vi "HAL process.vi"   [LabVIEW 2016]
uses:
  <vilib>/Plasmionique/MB Master/MB_Master/MB_Master.lvclass
  PLC/PLC.lvlib
types:
  T1 = cluster{"SYSTEM Interface":cluster{"运行模式":enum16{"维护模式", "常规模式", "应急模式", "质控模式"}, "站点类型":enum16{"一体站", "固定站"}, "CODMn类型":enum16{"PLC版", "单片机版"}, "总磷总氮类型":enum16{"单模块", "二合一模块"}}, "Pump Interface":cluster{"Pump MB session in":refnum<class "MB_Master.lvclass">}, "NH3N Interface":cluster{"NH3N session in":refnum<class "MB_Master.lvclass">, "氨氮自动测试量程配置":cluster{"水样测试量程模式":enum16{"H", "L", "AUTO"}, "空白核查量程模式":enum16{"H", "L", "AUTO"}, "跨度核查量程模式":enum16{"H", "L", "AUTO"}, "加标回收量程模式":enum16{"H", "L", "AUTO"}}}, "TP Interface":cluster{"TP MB session in":refnum<class "MB_Master.lvclass">, "总磷自动测试量程配置":cluster{"水样测试量程模式":enum16{"H", "L", "AUTO"}, "空白核查量程模式":enum16{"H", "L", "AUTO"}, "跨度核查量程模式":enum16{"H", "L", "AUTO"}, "加标回收量程模式":enum16{"H", "L", "AUTO"}}}, "TN Interface":cluster{"TN MB session in":refnum<class "MB_Master.lvclass">, "总氮自动测试量程配置":cluster{"水样测试量程模式":enum16{"H", "L", "AUTO"}, "空白核查量程模式":enum16{"H", "L", "AUTO"}, "跨度核查量程模式":enum16{"H", "L", "AUTO"}, "加标回收量程模式":enum16{"H", "L", "AUTO"}}}, "CODMn Interface":cluster{"CODMn MB session in":refnum<class "MB_Master.lvclass">, "CODMn自动测试量程配置":cluster{"水样测试量程模式":enum16{"H", "L", "AUTO"}, "空白核查量程模式":enum16{"H", "L", "AUTO"}, "跨度核查量程模式":enum16{"H", "L", "AUTO"}, "加标回收量程模式":enum16{"H", "L", "AUTO"}}}, "CODCr Interface":cluster{"CODCr MB session in":refnum<class "MB_Master.lvclass">, "CODCr自动测试量程配置":cluster{"水样测试量程模式":enum16{"H", "L", "AUTO"}, "空白核查量程模式":enum16{"H", "L", "AUTO"}, "跨度核查量程模式":enum16{"H", "L", "AUTO"}, "加标回收量程模式":enum16{"H", "L", "AUTO"}}}, "PLC_CODMn Interface":cluster{"PLC版_CODMn状态":u16, "PLC版_CODMn测量数据区":cluster{"因子编码":u32, "单位":u16, "标样参考值":sgl, "水样数据时间":timestamp, "水样实测值":sgl, "水样数据标识":string, "标样数据时间":timestamp, "标样实测值":sgl, "标样数据标识":string, "空白数据时间":timestamp, "空白实测值":sgl, "空白数据标识":string, "零点核查数据时间":timestamp, "零点核查实测值":sgl, "零点核查数据标识":string, "跨度核查数据时间":timestamp, "跨度核查实测值":sgl, "跨度核查数据标识":string, "加标回收数据时间":timestamp, "加标回收实测值":sgl, "加标回收数据标识":string, "平行样数据时间":timestamp, "平行样实测值":sgl, "平行样数据标识":string}}}
  T2 = cluster{"水样测试量程模式":enum16{"H", "L", "AUTO"}, "空白核查量程模式":enum16{"H", "L", "AUTO"}, "跨度核查量程模式":enum16{"H", "L", "AUTO"}, "加标回收量程模式":enum16{"H", "L", "AUTO"}}
  T3 = cluster{"水样测试量程模式":enum16{"H", "L", "AUTO"}, "空白核查量程模式":enum16{"H", "L", "AUTO"}, "跨度核查量程模式":enum16{"H", "L", "AUTO"}, "加标回收量程模式":enum16{"H", "L", "AUTO"}, "标样核查量程模式":enum16{"H", "L", "AUTO"}}
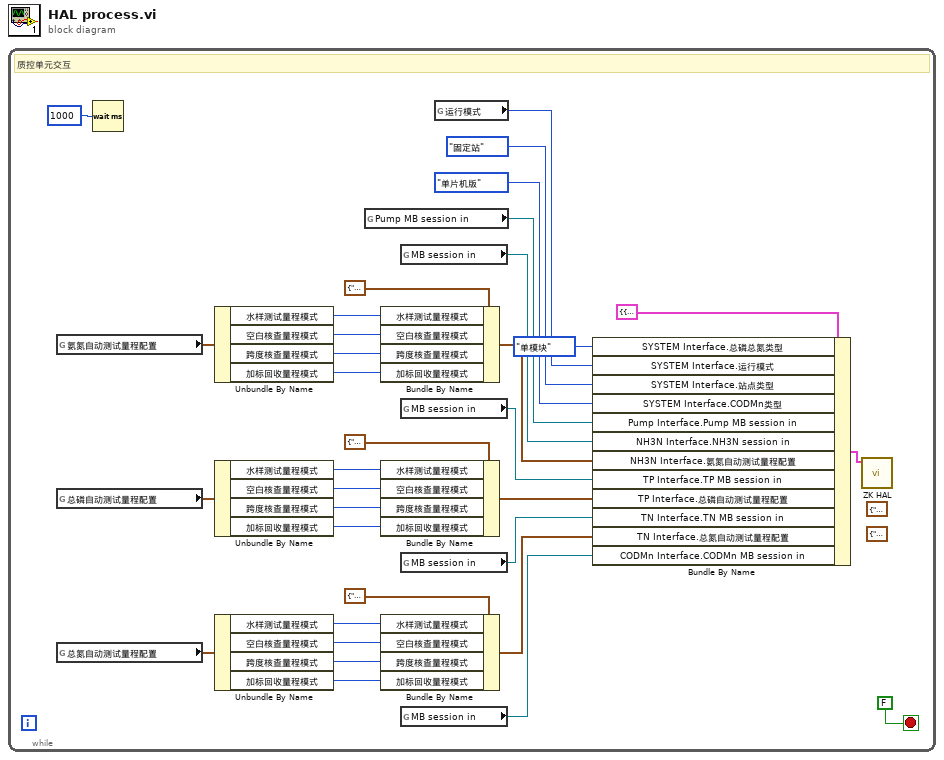
[diagram p0: block diagram]
diagram:
  n1 = while {
    stop <- FALSE stop-if-true
    (unwired) T2 {"水样测试量程模式"=enum."H", "空白核查量程模式"=enum."H", "跨度核查量程模式"=enum."H", "加标回收量程模式"=enum."H"} ("NH3N Interface.氨氮自动测试量程配置")
    (unwired) T2 {"水样测试量程模式"=enum."H", "空白核查量程模式"=enum."H", "跨度核查量程模式"=enum."H", "加标回收量程模式"=enum."H"} ("NH3N Interface.氨氮自动测试量程配置")
    # "质控单元交互"
    n2 = global read "总磷总氮断电保存全局变量.vi" "氨氮自动测试量程配置"() -> (w22:T3)
    n3 = global read "总磷总氮断电保存全局变量.vi" "总磷自动测试量程配置"() -> (w17:T3)
    n4 = global read "总磷总氮断电保存全局变量.vi" "总氮自动测试量程配置"() -> (w16:T3)
    n5 = Wait (ms)(milliseconds to wait=u32 1000 ("等待时间（毫秒）")) -> ()  [unwired: 1 out]
    n6 = Unbundle By Name(w22) -> ("水样测试量程模式"=w21:enum16{"H", "L", "AUTO"}, "空白核查量程模式"=w20:enum16{"H", "L", "AUTO"}, "跨度核查量程模式"=w19:enum16{"H", "L", "AUTO"}, "加标回收量程模式"=w18:enum16{"H", "L", "AUTO"})
    n7 = Unbundle By Name(w17) -> ("水样测试量程模式"=w13:enum16{"H", "L", "AUTO"}, "空白核查量程模式"=w12:enum16{"H", "L", "AUTO"}, "跨度核查量程模式"=w11:enum16{"H", "L", "AUTO"}, "加标回收量程模式"=w10:enum16{"H", "L", "AUTO"})
    n8 = Unbundle By Name(w16) -> ("水样测试量程模式"=w9:enum16{"H", "L", "AUTO"}, "空白核查量程模式"=w8:enum16{"H", "L", "AUTO"}, "跨度核查量程模式"=w7:enum16{"H", "L", "AUTO"}, "加标回收量程模式"=w6:enum16{"H", "L", "AUTO"})
    n9 = global read "采配水全局变量.vi" "Pump MB session in"() -> (w26:refnum<class "MB_Master.lvclass">)
    n10 = Bundle By Name(cluster=T2 {"水样测试量程模式"=enum."H", "空白核查量程模式"=enum."H", "跨度核查量程模式"=enum."H", "加标回收量程模式"=enum."H"} ("NH3N Interface.氨氮自动测试量程配置"), "水样测试量程模式"=w21, "空白核查量程模式"=w20, "跨度核查量程模式"=w19, "加标回收量程模式"=w18) -> (w23:T2)
    n11 = Bundle By Name(cluster=T2 {"水样测试量程模式"=enum."H", "空白核查量程模式"=enum."H", "跨度核查量程模式"=enum."H", "加标回收量程模式"=enum."H"} ("NH3N Interface.氨氮自动测试量程配置"), "水样测试量程模式"=w13, "空白核查量程模式"=w12, "跨度核查量程模式"=w11, "加标回收量程模式"=w10) -> (w5:T2)
    n12 = Bundle By Name(cluster=T2 {"水样测试量程模式"=enum."H", "空白核查量程模式"=enum."H", "跨度核查量程模式"=enum."H", "加标回收量程模式"=enum."H"} ("NH3N Interface.氨氮自动测试量程配置"), "水样测试量程模式"=w9, "空白核查量程模式"=w8, "跨度核查量程模式"=w7, "加标回收量程模式"=w6) -> (w4:T2)
    n13 = global read "VAR总磷总氮全局变量.vi" "MB session in"() -> (w29:refnum<class "MB_Master.lvclass">)
    n14 = global read "VAR总磷总氮全局变量.vi" "MB session in"() -> (w28:refnum<class "MB_Master.lvclass">)
    n15 = global read "VAR总磷总氮全局变量.vi" "MB session in"() -> (w27:refnum<class "MB_Master.lvclass">)
    n16 = global read "VARCODMn全局变量.vi" "MB session in"() -> (w25:refnum<class "MB_Master.lvclass">)
    n17 = global read "系统设置全局变量.vi" "运行模式"() -> (w30:enum16{"维护模式", "常规模式", "应急模式", "质控模式"})
    n18 = Bundle By Name(cluster=T1 {"SYSTEM Interface"={"运行模式"=enum."维护模式", "站点类型"=enum."一体站", "CODMn类型"=enum."PLC版", "总磷总氮类型"=enum."单模块"}, "Pump Interface"={"Pump MB session in"=refnum}, "NH3N Interface"={"NH3N session in"=refnum, "氨氮自动测试量程配置"={"水样测试量程模式"=enum."AUTO", "空白核查量程模式"=enum."AUTO", "跨度核查量程模式"=enum."AUTO", "加标回收量程模式"=enum."AUTO"}}, "TP Interface"={"TP MB session in"=refnum, "总磷自动测试量程配置"={"水样测试量程模式"=enum."AUTO", "空白核查量程模式"=enum."AUTO", "跨度核查量程模式"=enum."AUTO", "加标回收量程模式"=enum."AUTO"}}, "TN Interface"={"TN MB session in"=refnum, "总氮自动测试量程配置"={"水样测试量程模式"=enum."AUTO", "空白核查量程模式"=enum."AUTO", "跨度核查量程模式"=enum."AUTO", "加标回收量程模式"=enum."AUTO"}}, "CODMn Interface"={"CODMn MB session in"=refnum, "CODMn自动测试量程配置"={"水样测试量程模式"=enum."AUTO", "空白核查量程模式"=enum."AUTO", "跨度核查量程模式"=enum."AUTO", "加标回收量程模式"=enum."AUTO"}}, "CODCr Interface"={"CODCr MB session in"=refnum, "CODCr自动测试量程配置"={"水样测试量程模式"=enum."AUTO", "空白核查量程模式"=enum."AUTO", "跨度核查量程模式"=enum."AUTO", "加标回收量程模式"=enum."AUTO"}}, "PLC_CODMn Interface"={"PLC版_CODMn状态"=0, "PLC版_CODMn测量数据区"={"因子编码"=0, "单位"=0, "标样参考值"=0.0, "水样数据时间"=timestamp(0 s since 1904-01-01), "水样实测值"=0.0, "水样数据标识"="", "标样数据时间"=timestamp(0 s since 1904-01-01), "标样实测值"=0.0, "标样数据标识"="", "空白数据时间"=timestamp(0 s since 1904-01-01), "空白实测值"=0.0, "空白数据标识"="", "零点核查数据时间"=timestamp(0 s since 1904-01-01), "零点核查实测值"=0.0, "零点核查数据标识"="", "跨度核查数据时间"=timestamp(0 s since 1904-01-01), "跨度核查实测值"=0.0, "跨度核查数据标识"="", "加标回收数据时间"=timestamp(0 s since 1904-01-01), "加标回收实测值"=0.0, "加标回收数据标识"="", "平行样数据时间"=timestamp(0 s since 1904-01-01), "平行样实测值"=0.0, "平行样数据标识"=""}}} ("Interface"), "SYSTEM Interface.总磷总氮类型"=enum16{"单模块", "二合一模块"}."单模块", "SYSTEM Interface.运行模式"=w30, "SYSTEM Interface.站点类型"=enum16{"一体站", "固定站"}."固定站", "SYSTEM Interface.CODMn类型"=enum16{"PLC版", "单片机版"}."单片机版", "Pump Interface.Pump MB session in"=w26, "NH3N Interface.NH3N session in"=w29, "NH3N Interface.氨氮自动测试量程配置"=w23, "TP Interface.TP MB session in"=w28, "TP Interface.总磷自动测试量程配置"=w5, "TN Interface.TN MB session in"=w27, "TN Interface.总氮自动测试量程配置"=w4, "CODMn Interface.CODMn MB session in"=w25) -> (w2:T1)
    n19 = call "ZK HAL.vi"("Interface"=w2) -> ()  [unwired: 11 in]
  }
